vi "Timestamp_with_milliseconds_newFGGA_splitmilliseconds.vi"(0 "Input Time":string="07:54:55.584 08/08/18") -> (4 "Output Time":string, 8 "Output split millisecond":string)   [LabVIEW 2014]
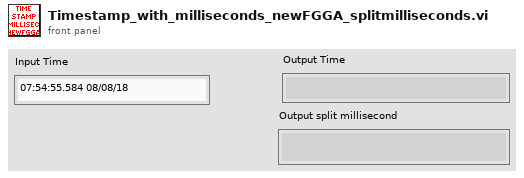
[diagram p1: front panel]
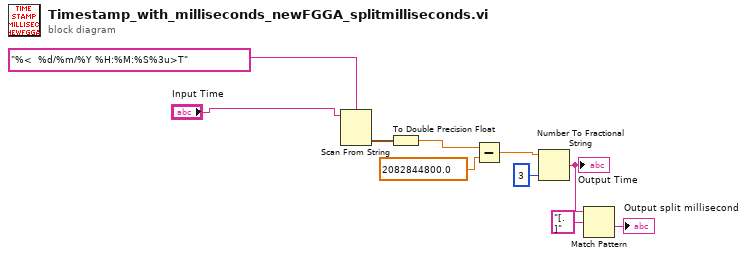
[diagram p0: block diagram]
diagram:
  n1 = Scan From String(format string="%<  %d/%m/%Y %H:%M:%S%3u>T", input string="Input Time") -> (output 1=w10:timestamp)  [unwired: 3 in, 3 out]
  n2 = To Double Precision Float(number=w10) -> (double precision float=w8:dbl)
  n3 = Subtract(x=w8, y=2082844800.0) -> (x-y=w7:dbl)
  n4 = Number To Fractional String(number=w7, precision (6)=i16 3) -> (F-format string=w3:string)  [unwired: 2 in]
  "Output Time" <- w3
  n5 = Match Pattern(string=w3, regular expression="[.]") -> (after substring=→"Output split millisecond":string)  [unwired: 1 in, 3 out]
